vi "parse.vi"(8 "error in (no error)":errorcluster, 10 "Frame":T1={"Data"=[], "WaitForTrigger"=FALSE, "WaitForRx"=0, "TriggerIRQ"=-1} {"Data" format="%02x"}, 11 "FrameParser in":refnum<class "FrameParser.lvclass">) -> (0 "error out":errorcluster, 3 "FrameParser out":refnum<class "FrameParser.lvclass">)   [LabVIEW 2015, in "FrameParser.lvclass"]
uses:
  FrameParser.lvclass
  Typedefs/Frame.ctl
  FrameParser.lvclass/FrameParser.ctl
  Typedefs/RTTypeDefs.lvlib
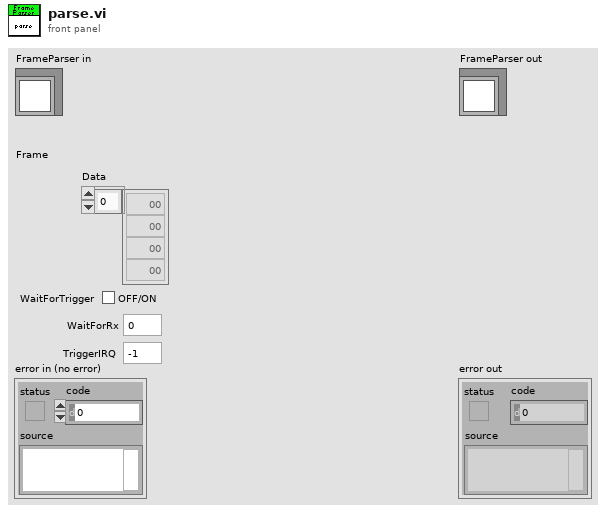
[diagram p1: front panel]
types:
  T1 = typedef "RTTypeDefs.lvlib/Frame.ctl" = cluster{"Data":u8[], "WaitForTrigger":bool, "WaitForRx":u16, "TriggerIRQ":i16}
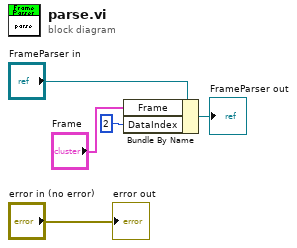
[diagram p0: block diagram]
diagram:
  n1 = Bundle By Name(cluster="FrameParser in", "Frame"="Frame", "DataIndex"=2) -> (→"FrameParser out":refnum<class "FrameParser.lvclass">)
  "error out" <- "error in (no error)"
